vi "TrioMotion_Test2.vi"() -> ()   [LabVIEW 2020]
uses:
  8fbe439c-06e5-460e-a560-e938ce784f44.vi
panel:
  out "Time Elapsed (s)":i32
  in  "Motion Tab":T1(tab)
  out "Axis 1 Endmove":dbl format="%.2g"
  out "Axis 1 Velocity":dbl format="%.2g"
  out "Axis 1 Position":dbl format="%.2g"
  out "Axis 0 Velocity":dbl format="%.2g"
  out "Axis 0 Endmove":dbl format="%.2g"
  out "Axis 0 Position":dbl format="%.2f"
  out "Axis 2 Position":dbl format="%#.2g"
  out "Axis 2 Endmove":dbl format="%#.2g"
  out "Axis 2 Velocity":dbl format="%#.2g"
  out "POWER OP":bool[](array[boolean])
  out "XY Graph":cluster{"X":dbl, "Y":dbl}[](graph)
  in  "Xmax":dbl=150.0 min=0.0 max=150.0 step=10.0
  in  "Xmin":dbl=-150.0 min=-150.0 max=0.0 step=10.0
  in  "Ymin":dbl=-150.0 min=-150.0 max=0.0 step=10.0
  in  "Ymax":dbl=150.0 min=0.0 max=150.0 step=10.0
  in  "Select Program":string(combo)="NONE"
  in  "Run Program":bool
  in  "Axis Enable":bool
  in  "Axis 0 Distance":dbl
  in  "Axis 1 Distance":dbl
  in  "Axis 2 Distance":dbl
  in  "Axis 0 Speed":dbl
  in  "Axis 1 Speed":dbl
  in  "Axis 2 Speed":dbl
  in  "Set Parameters 2":bool
  in  "Move":bool
  in  "Axis 1 Acc":dbl
  in  "Axis 0 Acc":dbl
  in  "Axis 2 Acc":dbl
  out "CommPort":fxp<+,3,3>
  in  "?":bool
  in  "Setup Tab":enum32{"SETUP", "POWER", "ERRORS"}(tab)
  out "IsOpen":bool
  in  "Connection":refnum<k7>(container)
  in  "Connect  to Controller":bool=TRUE
  out "Controller Type":string
  in  "Set Parameters":bool
  in  "Controller Connection Type":string(combo)="2"
  out "error out 2":errorcluster
  in  "error in (no error)":errorcluster
  out "Loop Time (us)":u32
  out "error out 3":errorcluster
  # "POSITION"
  # "ENDMOVE"
  # "VELOCITY"
  # "AXIS 0"
  # "AXIS 1"
  # "AXIS 2"
  # "SPEED SETTINGS"
  # "ACC SETTINGS"
  # "DISTANCE"
  # "CONNECTION SETTINGS"
  # "CONNECTION"
  # "LOGGING"
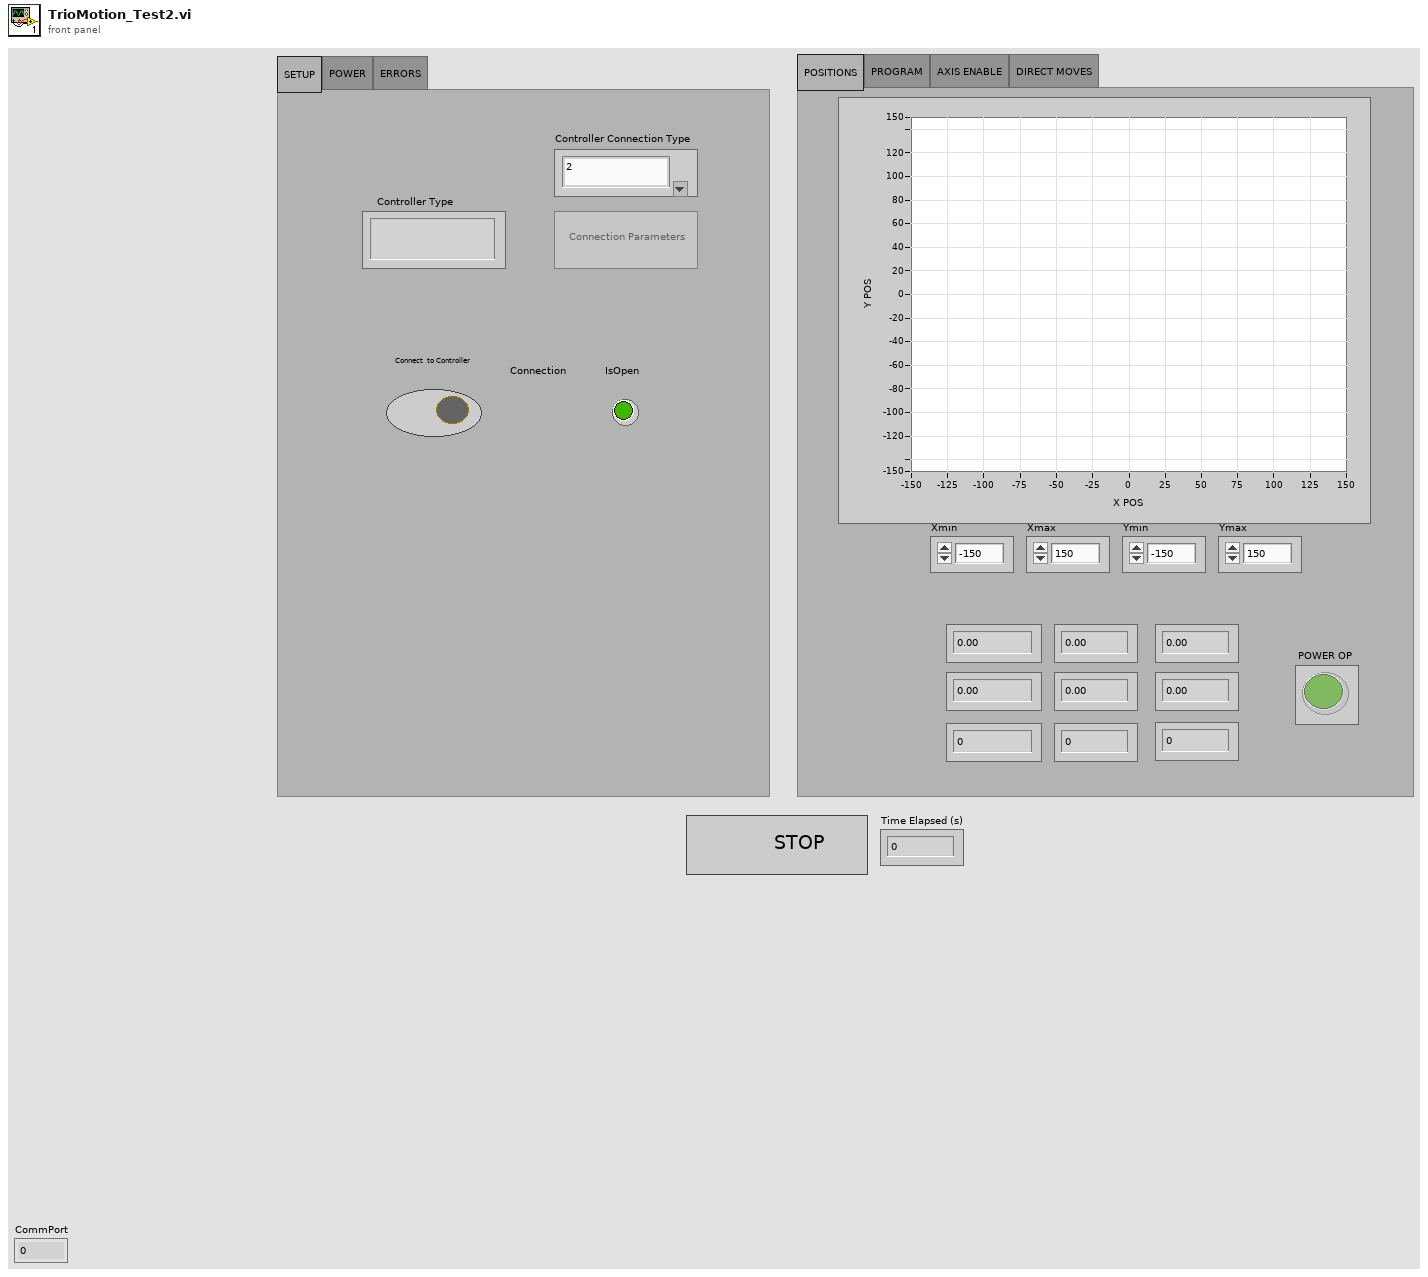
[diagram p1: front panel]
types:
  T1 = enum32{"POSITIONS", "PROGRAM", "AXIS ENABLE", "DIRECT MOVES"}
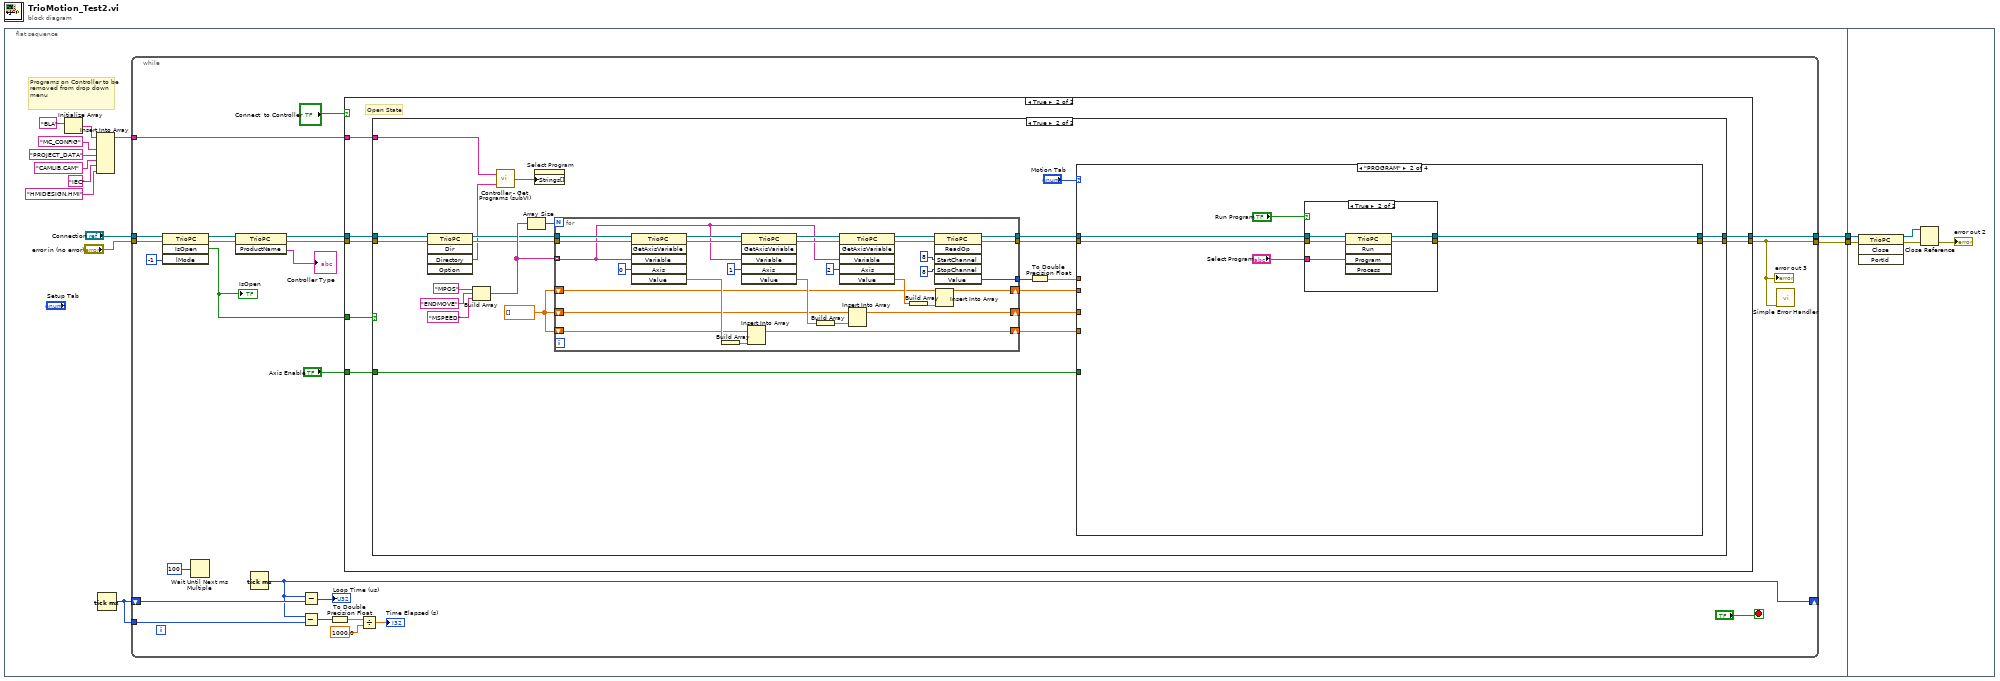
[diagram p0: block diagram]
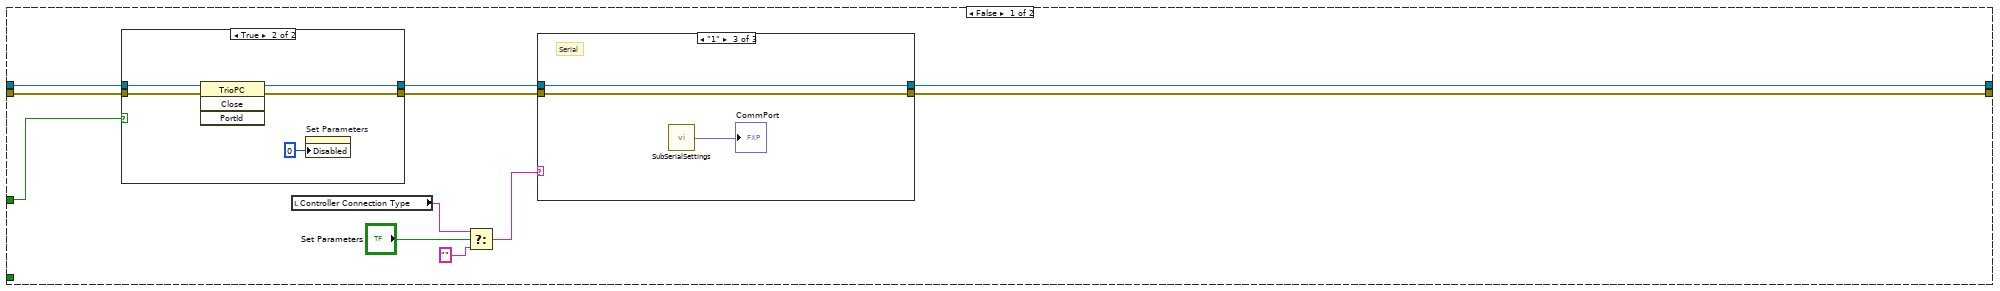
[diagram p2: hidden frame]
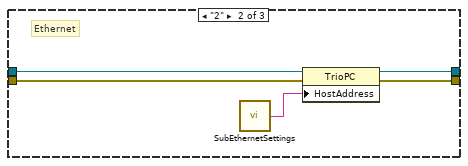
[diagram p5: hidden frame]
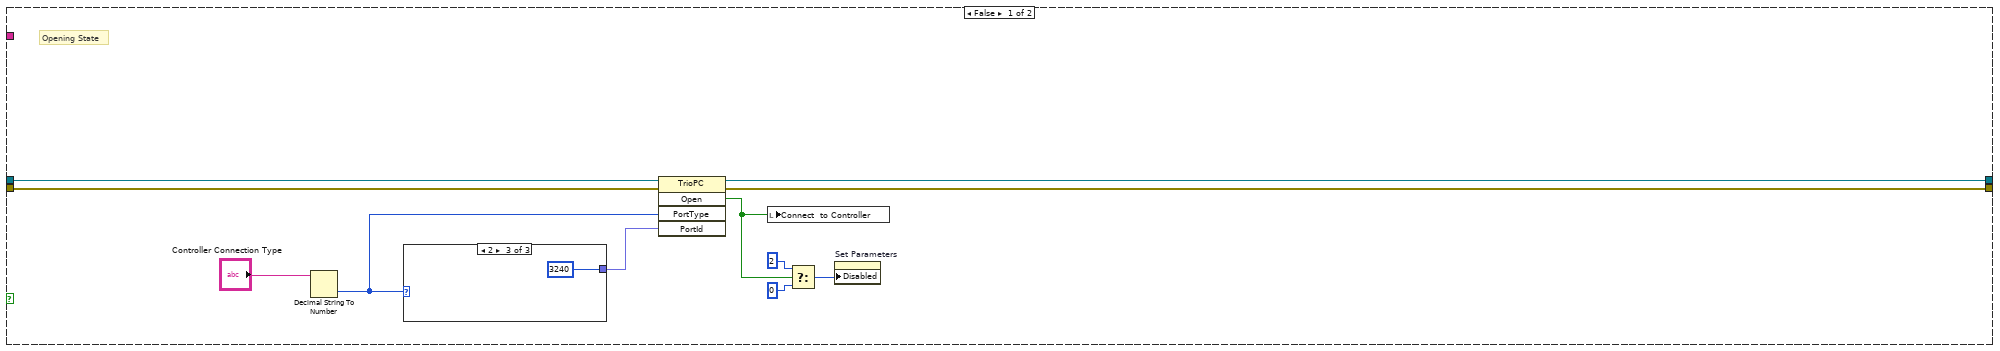
[diagram p6: hidden frame]
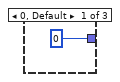
[diagram p7: hidden frame]
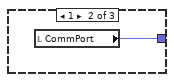
[diagram p8: hidden frame]
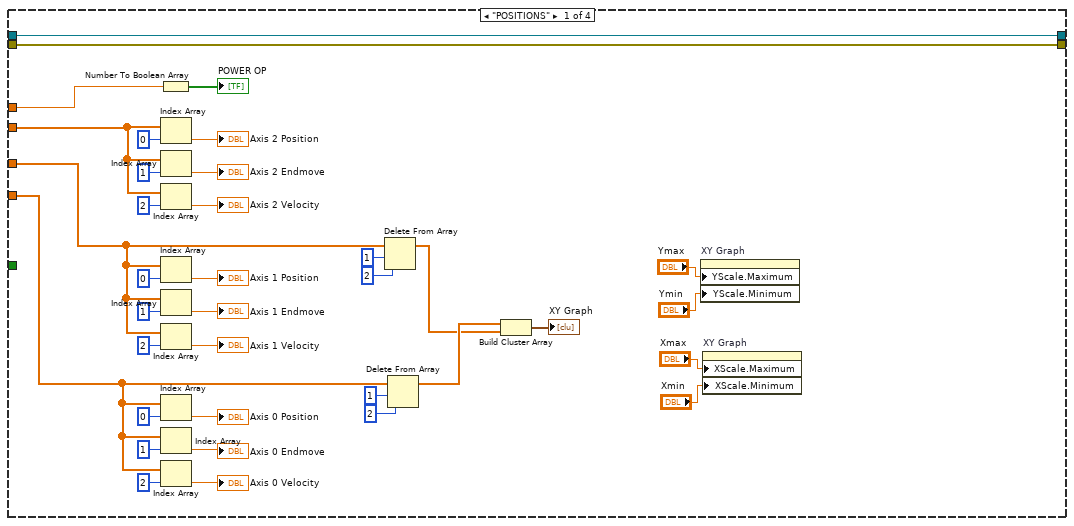
[diagram p9: hidden frame]
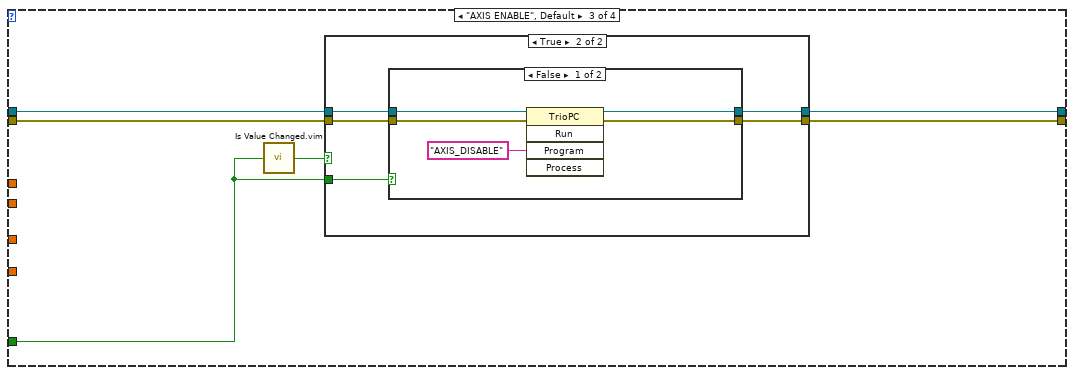
[diagram p11: hidden frame]
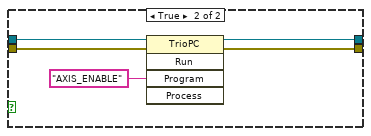
[diagram p13: hidden frame]
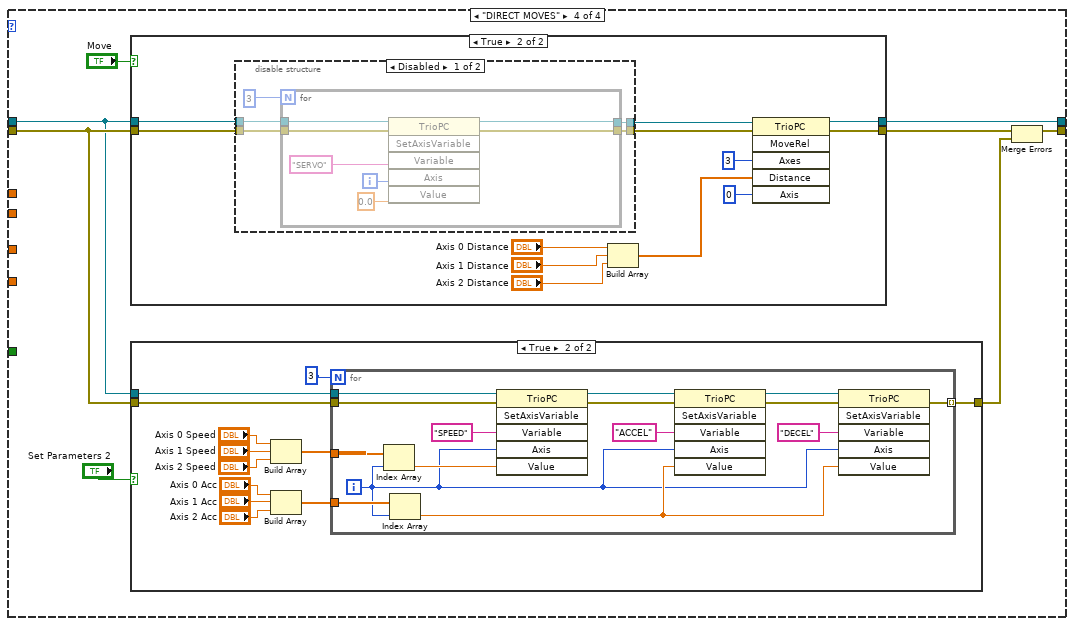
[diagram p14: hidden frame]
diagram:
  n1 = flat-sequence {
    tunnel: [w13] -> w2
    tunnel: [w12] -> w1
    tunnel: w2 -> [w281]
    tunnel: w1 -> [w280]
    frame #0 {
      # "Programs on Controller to be removed from drop down menu"
      n2 = Initialize Array("BLA" ("element")) -> (w11:string[])  [unwired: 1 in]
      n3 = Insert Into Array(array=w11, new element #1="MC_CONFIG" ("element"), new element #2="PROJECT_DATA" ("element"), new element #3="CAMLIB.CAM" ("element"), new element #4="IEC" ("element"), new element #5="HMIDESIGN.HMI") -> (w4:string[])  [unwired: 1 in]
      n4 = Tick Count (ms)() -> (millisecond timer value=w3:u32)
      n5 = while {
        tunnel: "Connection" -> [w34]
        tunnel: "error in (no error)" -> [w33]
        tunnel: [w30] -> w13
        tunnel: [w16] -> w12
        shift-right: [w19] -> _
        shift-left: w3 -> [w24]
        tunnel: w4 -> [w22]
        tunnel: w3 -> [w18]
        stop <- "?" stop-if-true
        n6 = invoke class="TrioPC" method="IsOpen"(reference=w34, error in=w33, "lMode"=-1) -> (reference out=w37:refnum<k7>, error out=w36:errorcluster, "IsOpen"=w31:bool)  [unwired: 1 in, 1 out]
        "IsOpen" <- w31
        n7 = Wait Until Next ms Multiple(millisecond multiple=u32 100) -> ()  [unwired: 1 out]
        n8 = invoke class="TrioPC" method="ProductName"(reference=w37, error in=w36) -> (reference out=w29:refnum<k7>, error out=w28:errorcluster, "ProductName"=→"Controller Type":string)  [unwired: 1 in]
        n9 = Tick Count (ms)() -> (millisecond timer value=w19:u32)
        n10 = Subtract(x=w19, y=w18) -> (x-y=w17:u32)
        n11 = Subtract(x=w19, y=w24) -> (x-y=→"Loop Time (us)":u32)
        n12 = To Double Precision Float(number=w17) -> (double precision float=w20:dbl)
        n13 = case shown="True" "Connect  to Controller" {
          tunnel: [w44 w74] -> w30
          tunnel: [w45 w73] -> w16
          tunnel: w31 -> [w41 w72]
          tunnel: w29 -> [w43 w71]
          tunnel: w28 -> [w42 w70]
          tunnel: w22 -> [_ w69]
          tunnel: "Axis Enable" -> [_ w68]
          frame False {
            n14 = case shown="True" w41 {
              tunnel: [w52 w57] -> w47
              tunnel: [w51 w56] -> w46
              tunnel: w43 -> [w52 w54]
              tunnel: w42 -> [w51 w53]
              frame False {
              }
              frame True {
                n15 = invoke class="TrioPC" method="Close"(reference=w54, error in=w53) -> (reference out=w57:refnum<k7>, error out=w56:errorcluster)  [unwired: 2 in, 2 out]
                n16 = property on="Set Parameters" class="Bool"("Disabled"=u8 0) -> ()  [unwired: 2 in, 2 out]
              }
            }
            n17 = local read "Controller Connection Type"() -> (w40:string)
            n18 = Select(t=w40, s="Set Parameters", f="") -> (s? t:f=w48:string)
            n19 = case shown="\"1\"" w48 {
              tunnel: w47 -> [w59 w62 w67]
              tunnel: w46 -> [w58 w61 w66]
              tunnel: [w59 w64 w67] -> w44
              tunnel: [w58 w63 w66] -> w45
              frame "", Default {
              }
              frame "2" {
                # "Ethernet"
                n20 = call "SubEthernetSettings.vi"() -> ("Ethernet IP Address 2"=w60:string)
                n21 = property class="TrioPC"(reference=w62, error in=w61, "HostAddress"=w60) -> (reference out=w64:refnum<k7>, error out=w63:errorcluster)
              }
              frame "1" {
                # "Serial"
                n22 = call "SubSerialSettings.vi"() -> ("CommPort"=→"CommPort":fxp<+,3,3>)
              }
            }
          }
          frame True {
            # "Open State"
            n23 = case shown="True" w72 {
              tunnel: [w79 w100] -> w74
              tunnel: [w84 w102] -> w73
              tunnel: w71 -> [w78 w106]
              tunnel: w70 -> [w77 w105]
              tunnel: w69 -> [_ w90]
              tunnel: w68 -> [_ w99]
              frame False {
                # "Opening State"
                n24 = Decimal String To Number(string="Controller Connection Type") -> (number=w75:i32)  [unwired: 2 in, 1 out]
                n25 = case shown="2" w75 {
                  tunnel: [i16 0 ("PortId") w87 i16 3240 ("PortId")] -> w85
                  frame 0, Default {
                  }
                  frame 1 {
                    n26 = local read "CommPort"() -> (w87:fxp<+,3,3>)
                  }
                  frame 2 {
                  }
                }
                n27 = invoke class="TrioPC" method="Open"(reference=w78, error in=w77, "PortType"=w75, "PortId"=w85) -> (reference out=w79:refnum<k7>, error out=w84:errorcluster, "Open"=w80:bool)  [unwired: 1 in, 2 out]
                n28 = local write "Connect  to Controller"(w80) -> ()
                n29 = Select(t=u8 2, s=w80, f=u8 0 ("Disabled")) -> (s? t:f=w81:u8)
                n30 = property on="Set Parameters" class="Bool"("Disabled"=w81) -> ()  [unwired: 2 in, 2 out]
              }
              frame True {
                w95 = dbl[] [] ("Array")
                n31 = invoke class="TrioPC" method="Dir"(reference=w106, error in=w105) -> (reference out=w97:refnum<k7>, error out=w96:errorcluster, "Directory"=w91:string)  [unwired: 3 in, 2 out]
                n32 = Build Array("MPOS", "ENDMOVE", "MSPEED") -> (w109:string[])
                n33 = call "Controller - Get Programs (subVI).vi"("Controller Directory"=w91, "Exclusion List"=w90) -> ("Programs List"=w89:string[])
                n34 = Array Size(array=w109) -> (size(s)=w110:i32)
                n35 = property on="Select Program" class="CmbBox"("Strings[]"=w89) -> ()  [unwired: 2 in, 2 out]
                n36 = for {
                  N: w110 -> [_]
                  shift-right: [w139] -> w94
                  shift-left: w95 -> [w130]
                  tunnel: [w138] -> w103
                  tunnel: [w135] -> w107
                  shift-right: [w129] -> w93
                  shift-left: w95 -> [w113]
                  tunnel: [w124] -> w101
                  tunnel: w97 -> [w126]
                  tunnel: w96 -> [w125]
                  tunnel: w109 -> [w114] mode=indexing
                  shift-right: [w116] -> w98
                  shift-left: w95 -> [w115]
                  n37 = invoke class="TrioPC" method="GetAxisVariable"(reference=w126, error in=w125, "Variable"=w114, "Axis"=i16 0) -> (reference out=w128:refnum<k7>, error out=w127:errorcluster, "Value"=w141:dbl)  [unwired: 2 in, 3 out]
                  n38 = Build Array(w141) -> (w140:dbl[])
                  n39 = invoke class="TrioPC" method="GetAxisVariable"(reference=w128, error in=w127, "Variable"=w114, "Axis"=i16 1) -> (reference out=w123:refnum<k7>, error out=w121:errorcluster, "Value"=w132:dbl)  [unwired: 2 in, 3 out]
                  n40 = Insert Into Array(array=w130, new element=w140) -> (w139:dbl[])  [unwired: 1 in]
                  n41 = Build Array(w132) -> (w131:dbl[])
                  n42 = invoke class="TrioPC" method="GetAxisVariable"(reference=w123, error in=w121, "Variable"=w114, "Axis"=i16 2) -> (reference out=w122:refnum<k7>, error out=w120:errorcluster, "Value"=w117:dbl)  [unwired: 2 in, 3 out]
                  n43 = Insert Into Array(array=w113, new element=w131) -> (w129:dbl[])  [unwired: 1 in]
                  n44 = Build Array(w117) -> (w118:dbl[])
                  n45 = invoke class="TrioPC" method="ReadOp"(reference=w122, error in=w120, "StartChannel"=i16 8, "StopChannel"=i16 8) -> (reference out=w124:refnum<k7>, error out=w138:errorcluster, "Value"=w135:i32)  [unwired: 2 in, 3 out]
                  n46 = Insert Into Array(array=w115, new element=w118) -> (w116:dbl[])  [unwired: 1 in]
                }
                n47 = To Double Precision Float(number=w107) -> (double precision float=w104:dbl)
                n48 = case shown="\"PROGRAM\"" "Motion Tab" {
                  tunnel: w104 -> [w166 _ _ _]
                  tunnel: w103 -> [w172 w183 w195 w219]
                  tunnel: [w172 w182 w193 w215] -> w102
                  tunnel: w101 -> [w171 w181 w194 w218]
                  tunnel: [w171 w180 w192 w217] -> w100
                  tunnel: w99 -> [_ _ w191 _]
                  tunnel: w98 -> [w170 _ _ _]
                  tunnel: w94 -> [w143 _ _ _]
                  tunnel: w93 -> [w142 _ _ _]
                  frame "POSITIONS" {
                    n49 = Number To Boolean Array(number=w166) -> (Boolean array=→"POWER OP":bool[])
                    n50 = Index Array(array=w170, index=0) -> (element=→"Axis 2 Position":dbl)
                    n51 = Index Array(array=w170, index=1) -> (element=→"Axis 2 Endmove":dbl)
                    n52 = Index Array(array=w170, index=2) -> (element=→"Axis 2 Velocity":dbl)
                    n53 = Index Array(array=w142, index=0) -> (element=→"Axis 1 Position":dbl)
                    n54 = Index Array(array=w142, index=1) -> (element=→"Axis 1 Endmove":dbl)
                    n55 = Index Array(array=w142, index=2) -> (element=→"Axis 1 Velocity":dbl)
                    n56 = Index Array(array=w143, index=0) -> (element=→"Axis 0 Position":dbl)
                    n57 = Index Array(array=w143, index=1) -> (element=→"Axis 0 Endmove":dbl)
                    n58 = Index Array(array=w143, index=2) -> (element=→"Axis 0 Velocity":dbl)
                    n59 = Delete From Array(array=w142, length=1, index=2) -> (array with subset deleted=w145:dbl[])  [unwired: 1 out]
                    n60 = Delete From Array(array=w143, length=1, index=2) -> (array with subset deleted=w164:dbl[])  [unwired: 1 out]
                    n61 = Build Cluster Array(w164, w145) -> (→"XY Graph":cluster{dbl, dbl}[])
                    n62 = property on="XY Graph" class="XYGraph (strict)"("YScale.Maximum"="Ymax", "YScale.Minimum"="Ymin") -> ()  [unwired: 2 in, 2 out]
                    n63 = property on="XY Graph" class="XYGraph (strict)"("XScale.Maximum"="Xmax", "XScale.Minimum"="Xmin") -> ()  [unwired: 2 in, 2 out]
                  }
                  frame "PROGRAM" {
                    n64 = case shown="True" "Run Program" {
                      tunnel: "Select Program" -> [_ w190]
                      tunnel: w183 -> [w185 w189]
                      tunnel: [w185 w188] -> w182
                      tunnel: w181 -> [w184 w187]
                      tunnel: [w184 w186] -> w180
                      frame False {
                      }
                      frame True {
                        n65 = invoke class="TrioPC" method="Run"(reference=w187, error in=w189, "Program"=w190) -> (reference out=w186:refnum<k7>, error out=w188:errorcluster)  [unwired: 2 in, 3 out]
                      }
                    }
                  }
                  frame "AXIS ENABLE", Default {
                    n66 = call "Is Value Changed.vim"("value"=w191) -> ("changed or first call?"=w196:bool)
                    n67 = case shown="True" w196 {
                      tunnel: [w198 w203] -> w193
                      tunnel: w195 -> [w198 w202]
                      tunnel: w194 -> [w197 w201]
                      tunnel: [w197 w200] -> w192
                      tunnel: w191 -> [_ w199]
                      frame False {
                      }
                      frame True {
                        n68 = case shown="False" w199 {
                          tunnel: [w208 w213] -> w203
                          tunnel: w202 -> [w207 w212]
                          tunnel: w201 -> [w206 w211]
                          tunnel: [w205 w210] -> w200
                          frame False {
                            n69 = invoke class="TrioPC" method="Run"(reference=w206, error in=w207, "Program"="AXIS_DISABLE") -> (reference out=w205:refnum<k7>, error out=w208:errorcluster)  [unwired: 2 in, 3 out]
                          }
                          frame True {
                            n70 = invoke class="TrioPC" method="Run"(reference=w211, error in=w212, "Program"="AXIS_ENABLE") -> (reference out=w210:refnum<k7>, error out=w213:errorcluster)  [unwired: 2 in, 3 out]
                          }
                        }
                      }
                    }
                  }
                  frame "DIRECT MOVES" {
                    n71 = case shown="True" "Move" {
                      tunnel: w219 -> [w222 w235]
                      tunnel: w218 -> [w223 w234]
                      tunnel: [w223 w225] -> w217
                      tunnel: [w222 w224] -> w216
                      frame False {
                      }
                      frame True {
                        n72 = disable-structure shown="Disabled" {
                          disable-tunnel: w235 -> [w240 w248]
                          disable-tunnel: w234 -> [w239 w249]
                          disable-tunnel: [w238 w249] -> w233
                          disable-tunnel: [w237 w248] -> w232
                          frame Disabled {
                            n73 = for {
                              N: 3 -> [_]
                              tunnel: w239 -> [w246]
                              tunnel: [w241] -> w238
                              tunnel: w240 -> [w247]
                              tunnel: [w243] -> w237
                              i -> [w242]
                              n74 = invoke class="TrioPC" method="SetAxisVariable"(reference=w246, error in=w247, "Variable"="SERVO", "Axis"=w242, "Value"=0.0) -> (reference out=w241:refnum<k7>, error out=w243:errorcluster)  [unwired: 1 in, 4 out]
                            }
                          }
                          frame Enabled {
                          }
                        }
                        n75 = Build Array("Axis 0 Distance", "Axis 1 Distance", "Axis 2 Distance") -> (w229:dbl[])
                        n76 = invoke class="TrioPC" method="MoveRel"(reference=w233, error in=w232, "Axes"=i16 3, "Distance"=w229, "Axis"=0) -> (reference out=w225:refnum<k7>, error out=w224:errorcluster)  [unwired: 1 in, 4 out]
                      }
                    }
                    n77 = case shown="True" "Set Parameters 2" {
                      tunnel: w219 -> [_ w255]
                      tunnel: w218 -> [_ w254]
                      tunnel: [_ w250] -> w214
                      frame False {
                      }
                      frame True {
                        n78 = Build Array("Axis 0 Speed", "Axis 1 Speed", "Axis 2 Speed") -> (w258:dbl[])
                        n79 = Build Array("Axis 0 Acc", "Axis 1 Acc", "Axis 2 Acc") -> (w257:dbl[])
                        n80 = for {
                          N: 3 -> [_]
                          tunnel: w258 -> [w275]
                          tunnel: w257 -> [w274]
                          tunnel: w254 -> [w270]
                          tunnel: w255 -> [w269]
                          tunnel: [w262] -> w250 mode=indexing
                          i -> [w271]
                          n81 = Index Array(array=w275, index=w271) -> (element=w273:dbl)
                          n82 = Index Array(array=w274, index=w271) -> (element=w272:dbl)
                          n83 = invoke class="TrioPC" method="SetAxisVariable"(reference=w270, error in=w269, "Variable"="SPEED", "Axis"=w271, "Value"=w273) -> (reference out=w268:refnum<k7>, error out=w267:errorcluster)  [unwired: 1 in, 4 out]
                          n84 = invoke class="TrioPC" method="SetAxisVariable"(reference=w268, error in=w267, "Variable"="ACCEL", "Axis"=w271, "Value"=w272) -> (reference out=w266:refnum<k7>, error out=w265:errorcluster)  [unwired: 1 in, 4 out]
                          n85 = invoke class="TrioPC" method="SetAxisVariable"(reference=w266, error in=w265, "Variable"="DECEL", "Axis"=w271, "Value"=w272) -> (error out=w262:errorcluster)  [unwired: 1 in, 5 out]
                        }
                      }
                    }
                    n86 = Merge Errors(w216, w214) -> (w215:errorcluster)
                  }
                }
              }
            }
          }
        }
        "error out 3" <- w16
        n87 = Divide(x=w20, y=1000.0) -> (x/y=→"Time Elapsed (s)":dbl)
        n88 = call <vilib>:"Simple Error Handler.vi"("error in (no error)"=w16) -> ()  [unwired: 4 in, 5 out]
      }
    }
    frame #1 {
      n89 = invoke class="TrioPC" method="Close"(reference=w281, error in=w280) -> (reference out=w277:refnum<k7>, error out=w279:errorcluster)  [unwired: 2 in, 2 out]
      n90 = Close Reference(reference=w277, error in (no error)=w279) -> (error out=→"error out 2":errorcluster)
    }
  }
